vi "MTS_ScannerXYZToImageXY.vi"(2 "Axis":enum32{"x-y", "x-z", "y-z"}(ring), 3 "Scanner XYZ":T1) -> (0 "Image Y":dbl, 1 "Image X":dbl)   [LabVIEW 2013]
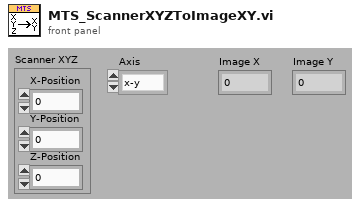
[diagram p1: front panel]
types:
  T1 = cluster{"X-Position":dbl, "Y-Position":dbl, "Z-Position":dbl}
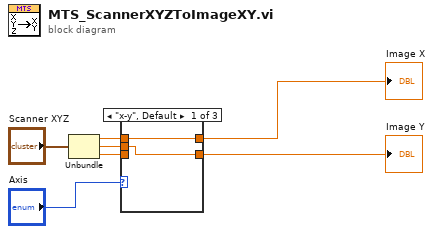
[diagram p0: block diagram]
diagram:
  n1 = Unbundle("Scanner XYZ") -> ("X-Position"=w3:dbl, "Y-Position"=w4:dbl, "Z-Position"=w5:dbl)
  n2 = case shown="\"x-y\", Default" "Axis" {
    tunnel: w3 -> [w9 w11 _]
    tunnel: w4 -> [w8 _ w13]
    tunnel: w5 -> [_ w10 w12]
    tunnel: [w9 w11 w13] -> w6
    tunnel: [w8 w10 w12] -> w7
    frame "x-y", Default {
    }
    frame "x-z" {
    }
    frame "y-z" {
    }
  }
  "Image Y" <- w7
  "Image X" <- w6
